vi "test Parameter Add-Find-Remove.vi"(8 "error in":errorcluster, 11 "TestCase in":refnum<class "Scripting.lvclass">) -> (0 "error out":errorcluster, 3 "TestCase out":refnum<class "Scripting.lvclass">)   [LabVIEW 2020, in "Scripting.lvclass"]
uses:
  Scripting.lvclass
  <vilib>/addons/_JKI Toolkits/VI Tester/TestCase.llb/TestCase.lvclass
  Scripting/AIM/AIM ARINC 429 Scripting.lvlib
  Shared/Direction.ctl
  <vilib>/NI VeriStand/Custom Device API/Custom Device Item Ref.ctl
  <vilib>/NI VeriStand/Custom Device API/Custom Device API.lvlib
  Shared/SDI.ctl
  <vilib>/NI/NI VeriStand Encoding and Decoding/Encoding.ctl
  <vilib>/NI/NI VeriStand Encoding and Decoding/Encoding and Decoding.lvlib
  Shared/Parameter Definition.ctl
  C:/Program Files (x86)/National Instruments/LabVIEW 2020/vi.lib/addons/_JKI Toolkits/VI Tester/TestCase.llb/TestCase.lvclass
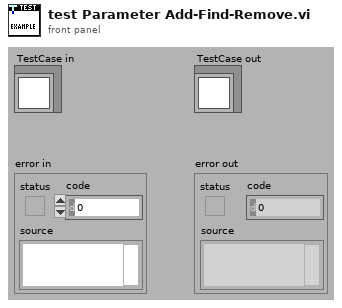
[diagram p1: front panel]
types:
  T1 = cluster{"SDI":bool, "SSM":bool, "Parity":bool, "Timestamp":bool}
  T2 = typedef "Parameter Definition.ctl" = cluster{"start index":i32, "size":i32, "encoding":T3, "signed":bool, "scale multiplier":dbl, "scale offset":dbl}
  T3 = typedef "Encoding and Decoding.lvlib/Encoding.ctl" = enum16{"BNR", "BCD", "Discrete"}
  T4 = typedef "Direction.ctl" = enum16{"Rx", "Tx"}
  T5 = typedef "Custom Device API.lvlib/Custom Device Item Ref.ctl" = u64
  T6 = cluster{"name":string, "unit":string, "default value":dbl}
  T7 = typedef "SDI.ctl" = i32
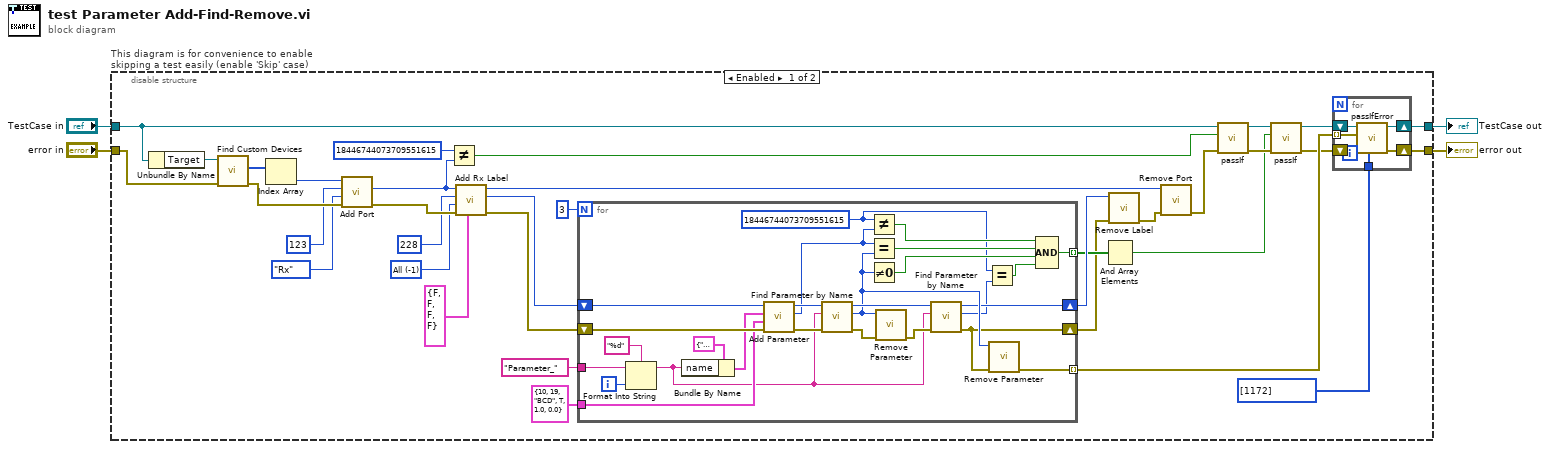
[diagram p0: block diagram]
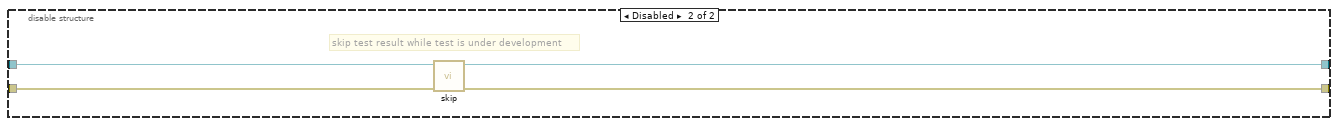
[diagram p2: hidden frame]
diagram:
  n1 = disable-structure "This diagram is for convenience to enable skipping a test easily (enable 'Skip' case)" shown="Enabled" {
    disable-tunnel: "TestCase in" -> [w36 w75]
    disable-tunnel: [w8 w73] -> w1
    disable-tunnel: [w9 w74] -> w3
    disable-tunnel: "error in" -> [w38 w72]
    frame Enabled {
      w31 = T7 -1 items=["All"=-1, "0 (b00)"=0, "1 (b01)"=1, "2 (b10)"=2, "3 (b11)"=3] ("SDI value")
      n2 = Unbundle By Name(w36) -> ("Target"=w39:refnum<k24>)
      n3 = call "Find Custom Devices.vi"("error in"=w38, "target in"=w39) -> ("error out"=w29:errorcluster, "AIM ARINC 429 custom devices"=w37:u64[])  [unwired: 7 in, 1 out]
      n4 = Index Array(array=w37) -> (element=w30:u64)  [unwired: 1 in]
      n5 = call "Add Port.vi"("error in"=w29, "direction"=Direction."Rx", "port number"=u16 123, "AIM ARINC 429 custom device in"=w30) -> ("error out"=w35:errorcluster, "port"=w24:T5)  [unwired: 5 in, 1 out]
      n6 = Not Equal?(x=T5 18446744073709551615 ("custom device ref out"), y=w24) -> (x != y?=w25:bool)
      n7 = call "Add Rx Label.vi"("create channels"=T1 {"SDI"=FALSE, "SSM"=FALSE, "Parity"=FALSE, "Timestamp"=FALSE}, "error in"=w35, "SDI value"=w31, "label value"=u32 228, "port in"=w24) -> ("error out"=w18:errorcluster, "label"=w20:T5, "port out"=w34:T5)  [unwired: 4 in]
      n8 = for {
        N: 3 -> [_]
        shift-right: [w51] -> w19
        shift-left: w20 -> [w71]
        shift-right: [w48] -> w14
        shift-left: w18 -> [w65]
        tunnel: T2 {"start index"=10, "size"=19, "encoding"=enum."BCD", "signed"=TRUE, "scale multiplier"=1.0, "scale offset"=0.0} ("parameter definition") -> [w64]
        tunnel: "Parameter_" ("initial string") -> [w61]
        tunnel: [w52] -> w15 mode=indexing
        tunnel: [w47] -> w12 mode=indexing
        i -> [w62]
        w50 = T5 18446744073709551615 ("custom device ref out")
        n9 = Format Into String(format string="%d", initial string=w61, w62) -> (resulting string=w58:string)  [unwired: 1 in, 1 out]
        n10 = Bundle By Name(cluster=T6 {"name"="", "unit"="super units", "default value"=3.0} ("parameter"), "name"=w58) -> (w59:T6)
        n11 = call "Add Parameter.vi"("error in"=w65, "parameter encoding"=w64, "parameter definition"=w59, "label in"=w71) -> ("error out"=w66:errorcluster, "parameter"=w57:T5, "label out"=w70:T5)  [unwired: 5 in]
        n12 = call "Find Parameter by Name.vi"("error in"=w66, "parameter name"=w58, "label in"=w70) -> ("error out"=w67:errorcluster, "parameter ref"=w56:T5, "label out"=w68:T5)  [unwired: 5 in, 1 out]
        n13 = Not Equal?(x=w50, y=w57) -> (x != y?=w54:bool)
        n14 = Equal?(x=w57, y=w56) -> (x = y?=w55:bool)
        n15 = Not Equal To 0?(x=w56) -> (x != 0?=w53:bool)
        n16 = call "Remove Parameter.vi"("error in"=w67, "parameter"=w56) -> ("error out"=w69:errorcluster)  [unwired: 9 in]
        n17 = call "Find Parameter by Name.vi"("error in"=w69, "parameter name"=w58, "label in"=w68) -> ("error out"=w48:errorcluster, "parameter ref"=w46:T5, "label out"=w51:T5)  [unwired: 5 in, 1 out]
        n18 = Equal?(x=w50, y=w46) -> (x = y?=w49:bool)
        n19 = call "Remove Parameter.vi"("error in"=w48, "parameter"=w56) -> ("error out"=w47:errorcluster)  [unwired: 9 in]
        n20 = Compound Arithmetic op=AND(w54, w55, w53, w49) -> (w52:bool)
      }
      n21 = And Array Elements(Boolean array=w15) -> (logical AND=w13:bool)
      n22 = call "Remove Label.vi"("error in"=w14, "label"=w19) -> ("error out"=w23:errorcluster)  [unwired: 9 in]
      n23 = call "Remove Port.vi"("error in"=w23, "port"=w34) -> ("error out"=w6:errorcluster)  [unwired: 9 in]
      n24 = call-dynamic "passIf.vi"("error in (no error)"=w6, "pass"=w25, "TestCase in"=w36) -> ("error out"=w22:errorcluster, "TestCase out"=w33:refnum<class "Scripting.lvclass">)  [unwired: 7 in]
      n25 = call-dynamic "passIf.vi"("error in (no error)"=w22, "pass"=w13, "TestCase in"=w33) -> ("error out"=w10:errorcluster, "TestCase out"=w11:refnum<class "Scripting.lvclass">)  [unwired: 7 in]
      n26 = for {
        tunnel: w12 -> [w45] mode=indexing
        shift-right: [w42] -> w8
        shift-left: w11 -> [w43]
        shift-right: [w41] -> w9
        shift-left: w10 -> [w44]
        tunnel: i32[] [1172] ("passing error codes (default = any error code)") -> [w40]
        n27 = call-dynamic "passIfError.vi"("passing error codes (default = any error code)"=w40, "error in (no error)"=w44, "error"=w45, "TestCase in"=w43) -> ("error out"=w41:errorcluster, "TestCase out"=w42:refnum<class "Scripting.lvclass">)  [unwired: 6 in]
      }
    }
    frame Disabled {
      # "skip test result while test is under development"
      n28 = call <vilib>:"skip.vi"("error in (no error)"=w72, "TestCase in"=w75) -> ("error out"=w74:errorcluster, "TestCase out"=w73:refnum<class "Scripting.lvclass">)  [unwired: 8 in]
    }
  }
  "error out" <- w3
  "TestCase out" <- w1
